vi "Arms Test.vi"(11 "Pilot-CoPilot Gamepad Controls":T1) -> ()   [LabVIEW 2014]
uses:
  Subsystems VIs/Robot Control Outputs 2015.ctl
  <vilib>/Rock Robotics/WPI/Solenoid/WPI_SolenoidValue.ctl
  <vilib>/Rock Robotics/Network Tables/SD Write Boolean Array.vi
  Global Variables/Refnum Names.vi
  <vilib>/Rock Robotics/WPI/Solenoid/WPI_SolenoidSetEnum.vi
panel:
  # "CB = control board"
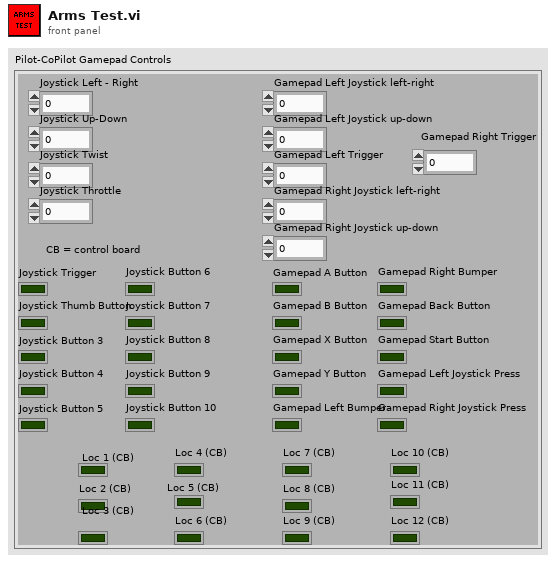
[diagram p1: front panel]
types:
  T1 = typedef "Robot Control Outputs 2015.ctl" = cluster{"Gamepad Left Joystick left-right":dbl, "Gamepad Left Joystick up-down":dbl, "Gamepad A Button":bool, "Gamepad B Button":bool, "Gamepad X Button":bool, "Gamepad Y Button":bool, "Gamepad Left Bumper":bool, "Gamepad Right Bumper":bool, "Gamepad Back Button":bool, "Gamepad Start Button":bool, "Gamepad Left Joystick Press":bool, "Gamepad Right Joystick Press":bool, "Joystick Trigger":bool, "Joystick Thumb Button":bool, "Joystick Button 3":bool, "Joystick Button 4":bool, "Joystick Button 5":bool, "Joystick Button 6":bool, "Joystick Button 7":bool, "Joystick Button 8":bool, "Joystick Button 9":bool, "Joystick Button 10":bool, "Gamepad Left Trigger":dbl, "Gamepad Right Joystick left-right":dbl, "Gamepad Right Joystick up-down":dbl, "Joystick Left - Right":dbl, "Joystick Up-Down":dbl, "Joystick Twist":dbl, "Joystick Throttle":dbl, "Loc 1 (CB)":bool, "Loc 4 (CB)":bool, "Gamepad Right Trigger":dbl, "Loc 2 (CB)":bool, "Loc 3 (CB)":bool, "Loc 5 (CB)":bool, "Loc 6 (CB)":bool, "Loc 7 (CB)":bool, "Loc 10 (CB)":bool, "Loc 8 (CB)":bool, "Loc 9 (CB)":bool, "Loc 11 (CB)":bool, "Loc 12 (CB)":bool}
  T2 = typedef "WPI_ServoDeviceRef.ctl" = cluster{"DeviceStatus":errorcluster, "Controller":T3, "PWM Channel":T4, "DeadBand":T5}
  T3 = typedef "FPGA_TypedefDigitalModule.ctl" = enum16{"Controller 1"}
  T4 = typedef "FPGA_DIOPWMChannel.ctl" = enum8{"PWM 0", "PWM 1", "PWM 2", "PWM 3", "PWM 4", "PWM 5", "PWM 6", "PWM 7", "PWM 8", "PWM 9", "PWM MXP 0", "PWM MXP 1", "PWM MXP 2", "PWM MXP 3", "PWM MXP 4", "PWM MXP 5", "PWM MXP 6", "PWM MXP 7", "PWM MXP 8", "PWM MXP 9", "Invalid"}
  T5 = typedef "WPI_PWMDeadband.ctl" = cluster{"Name":string, "maxPositivePwm":i32, "minPositivePwm":i32, "centerPwm":i32, "maxNegativePwm":i32, "minNegativePwm":i32, "angularRange":u16}
  T6 = typedef "WPI_SolenoidDevRef.ctl" = cluster{"DevStatus":errorcluster, "Pneumatics Control Module":u8, "Forward Solenoid Channel":T7, "Reverse Solenoid Channel":T7}
  T7 = typedef "WPI_SolenoidChannel.ctl" = enum8{"Solenoid 0", "Solenoid 1", "Solenoid 2", "Solenoid 3", "Solenoid 4", "Solenoid 5", "Solenoid 6", "Solenoid 7", "Invalid"}
  T8 = typedef "WPI_SolenoidValue.ctl" = enum16{"Off", "On", "Forward", "Reverse"}
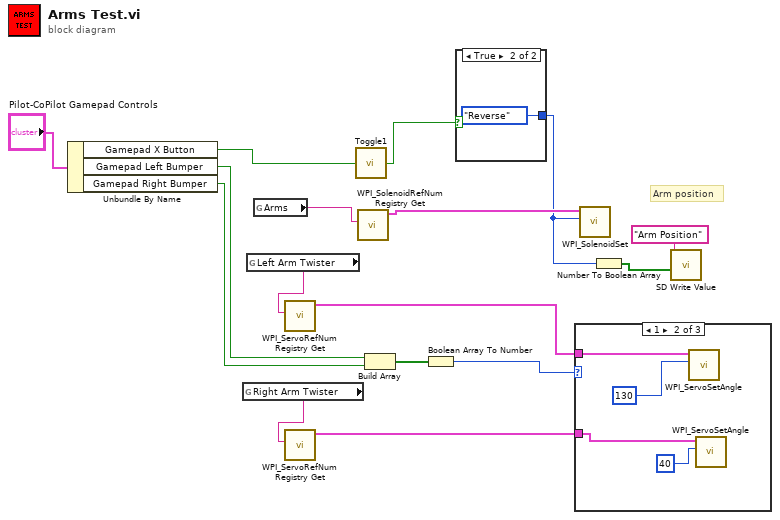
[diagram p0: block diagram]
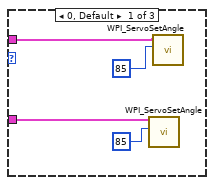
[diagram p2: hidden frame]
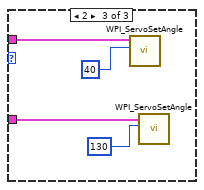
[diagram p3: hidden frame]
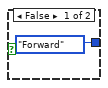
[diagram p4: hidden frame]
diagram:
  # "Arm position"
  n1 = Unbundle By Name("Pilot-CoPilot Gamepad Controls") -> ("Gamepad X Button"=w15:bool, "Gamepad Left Bumper"=w5:bool, "Gamepad Right Bumper"=w4:bool)
  n2 = global read "Refnum Names.vi" "Right Arm Twister"() -> (w2:string)
  n3 = global read "Refnum Names.vi" "Left Arm Twister"() -> (w11:string)
  n4 = global read "Refnum Names.vi" "Arms"() -> (w13:string)
  n5 = call <vilib>:"WPI_ServoRefNum Registry Get.vi"("refnum name"=w11) -> ("ServoDeviceRef"=w6:T2)  [unwired: 9 in, 1 out]
  n6 = call <vilib>:"WPI_ServoRefNum Registry Get.vi"("refnum name"=w2) -> ("ServoDeviceRef"=w1:T2)  [unwired: 9 in, 1 out]
  n7 = call "Toggle1.vi"("Boolean"=w15) -> ("Driver Switch 2"=w14:bool)
  n8 = call <vilib>:"WPI_SolenoidRefNum Registry Get.vi"("refnum name"=w13) -> ("SolenoidDevRef"=w12:T6)  [unwired: 9 in, 1 out]
  n9 = Build Array(w5, w4) -> (w3:bool[])
  n10 = Boolean Array To Number(Boolean array=w3) -> (number=w7:u32)
  n11 = case shown="True" w14 {
    tunnel: [WPI_SolenoidValue."Forward" ("Value") WPI_SolenoidValue."Reverse" ("Value")] -> w9
    frame False {
    }
    frame True {
    }
  }
  n12 = case shown="1" w7 {
    tunnel: w6 -> [w22 w26 w30]
    tunnel: w1 -> [w20 w23 w28]
    frame 0, Default {
      n13 = call <vilib>:"WPI_ServoSetAngle.vi"("Angle"=85, "ServoDeviceRef"=w20) -> ()  [unwired: 8 in, 2 out]
      n14 = call <vilib>:"WPI_ServoSetAngle.vi"("Angle"=85, "ServoDeviceRef"=w22) -> ()  [unwired: 8 in, 2 out]
    }
    frame 1 {
      n15 = call <vilib>:"WPI_ServoSetAngle.vi"("Angle"=130, "ServoDeviceRef"=w26) -> ()  [unwired: 8 in, 2 out]
      n16 = call <vilib>:"WPI_ServoSetAngle.vi"("Angle"=40, "ServoDeviceRef"=w23) -> ()  [unwired: 8 in, 2 out]
    }
    frame 2 {
      n17 = call <vilib>:"WPI_ServoSetAngle.vi"("Angle"=40, "ServoDeviceRef"=w30) -> ()  [unwired: 8 in, 2 out]
      n18 = call <vilib>:"WPI_ServoSetAngle.vi"("Angle"=130, "ServoDeviceRef"=w28) -> ()  [unwired: 8 in, 2 out]
    }
  }
  n19 = call-poly <vilib>:"WPI_SolenoidSet.vi"("Value"=w9, "SolenoidDevRef"=w12) -> ()  [unwired: 8 in, 2 out]
  n20 = Number To Boolean Array(number=w9) -> (Boolean array=w10:bool[])
  n21 = call-poly <vilib>:"SD Write Value.vi"("Boolean Array"=w10, "Name"="Arm Position") -> ()  [unwired: 8 in, 2 out]
